vi "Anritsu VNA Set IFBW.vi"(6 "Channel":i8=1 min=1 step=1, 7 "Anritsu VNA":T1, 8 "error in (no error)":errorcluster, 10 "IFBW, Hz (3000)":dbl=3000.0, 11 "VISA Resource Name":refnum<visa-resource-name>) -> (0 "error out":errorcluster, 3 "dup VISA Resource Name":refnum<visa-resource-name>)   [LabVIEW 2011]
doc: "This Vi for the HP8753B Network Analyzer is used to set averaging, smoothing, and the IF bandwidth."
uses:
  TypeDefs/Anritsu VNA Instrument Info.ctl
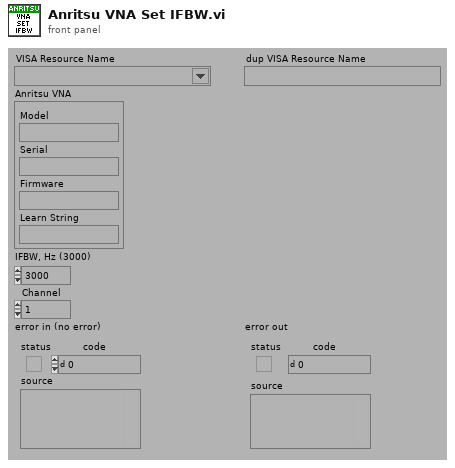
[diagram p1: front panel]
types:
  T1 = typedef "Anritsu VNA Instrument Info.ctl" = cluster{"Model":string, "Serial":string, "Firmware":string, "Learn String":string}
  T2 = typedef "Anritsu VNA Model.ctl" = enum16{"Not Supported", "37XXXX", "MS20XXX", "MS462XX", "MS464XX"}
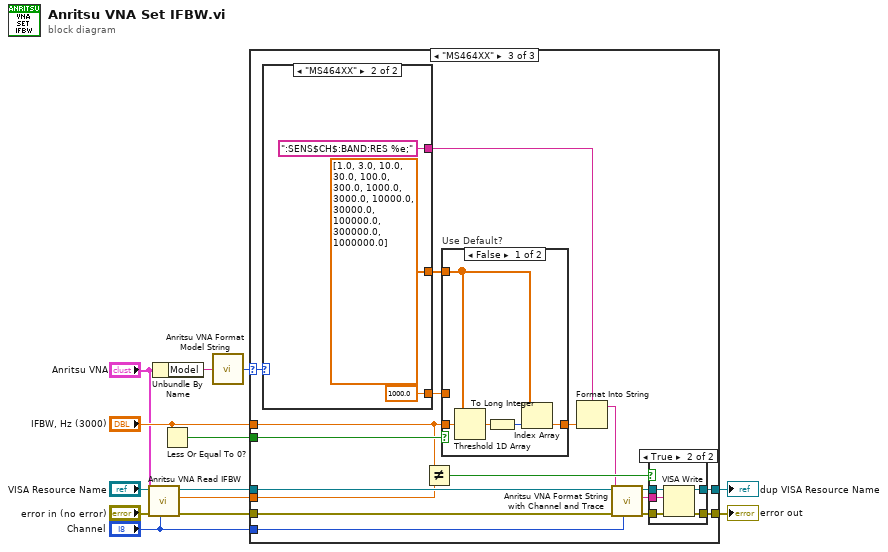
[diagram p0: block diagram]
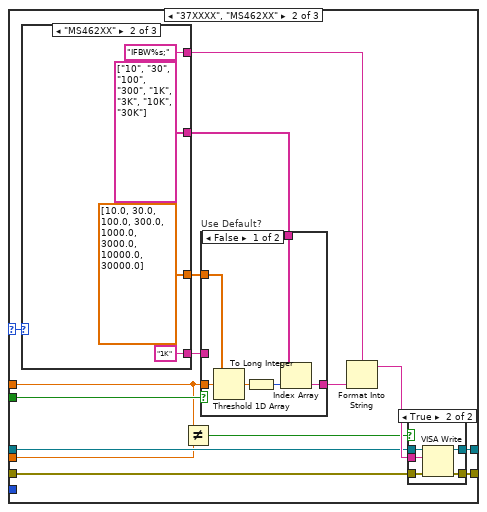
[diagram p3: hidden frame]
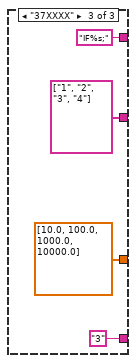
[diagram p6: hidden frame]
diagram:
  n1 = call "Anritsu VNA Read IFBW.vi"("Channel"="Channel", "Anritsu VNA"="Anritsu VNA", "error in (no error)"="error in (no error)", "VISA Resource Name"="VISA Resource Name") -> ("error out"=w8:errorcluster, "IFBW, Hz"=w7:dbl, "dup VISA Resource Name"=w9:refnum<visa-resource-name>)  [unwired: 5 out]
  n2 = Unbundle By Name("Anritsu VNA") -> ("Model"=w3:string)
  n3 = Less Or Equal To 0?(x="IFBW, Hz (3000)") -> (x <= 0?=w5:bool)
  n4 = call "Anritsu VNA Format Model String.vi"("Model"=w3) -> ("Model"=w2:T2)
  n5 = case shown="\"MS464XX\"" w2 {
    selector: w2 -> [_ w21 w60]
    tunnel: [w15 w30 w68] -> w13
    tunnel: [w14 w29 w67] -> w12
    tunnel: w9 -> [w14 w27 w66]
    tunnel: w8 -> [w15 w26 w65]
    tunnel: w7 -> [_ w24 w63]
    tunnel: "IFBW, Hz (3000)" -> [_ w17 w57]
    tunnel: w5 -> [_ w22 w61]
    tunnel: "Channel" -> [_ _ w53]
    frame "Not Supported", "MS20XXX" {
      # "The MS20XXX do not have the ability to set the IFBW."
    }
    frame "37XXXX", "MS462XX" {
      n6 = case shown="\"MS462XX\"" w21 {
        tunnel: [_ dbl[] [10.0, 30.0, 100.0, 300.0, 1000.0, 3000.0, 10000.0, 30000.0] dbl[] [10.0, 100.0, 1000.0, 10000.0]] -> w20
        tunnel: [_ "1K" "3"] -> w19
        tunnel: [_ string[] ["10", "30", "100", "300", "1K", "3K", "10K", "30K"] string[] ["1", "2", "3", "4"]] -> w18
        tunnel: [_ "IFBW%s;" "IF%s;"] -> w16
        frame "Not Supported", "MS20XXX", "MS464XX" {
        }
        frame "MS462XX" {
        }
        frame "37XXXX" {
        }
      }
      n7 = Not Equal?(x=w17, y=w24) -> (x != y?=w25:bool)
      n8 = case "Use Default?" shown="False" w22 {
        tunnel: w20 -> [w35 _]
        tunnel: w17 -> [w33 _]
        tunnel: [w32 w37] -> w23
        tunnel: w19 -> [_ w37]
        tunnel: w18 -> [w31 _]
        frame False {
          n9 = Threshold 1D Array(2:w33, 3:w35) -> (0:w36:dbl)  [unwired: 1 out]
          n10 = To Long Integer(number=w36) -> (32bit integer=w34:i32)
          n11 = Index Array(array=w31, index=w34) -> (element=w32:string)
        }
        frame True {
        }
      }
      n12 = Format Into String(format string=w16, w23) -> (resulting string=w28:string)  [unwired: 2 in, 1 out]
      n13 = case shown="True" w25 {
        tunnel: [w46 w52] -> w30
        tunnel: [w47 w51] -> w29
        tunnel: w28 -> [_ w50]
        tunnel: w27 -> [w47 w49]
        tunnel: w26 -> [w46 w48]
        frame False {
        }
        frame True {
          n14 = VISA Write(VISA resource name=w49, write buffer=w50, error in (no error)=w48) -> (VISA resource name out=w51:refnum<visa-resource-name>, error out=w52:errorcluster)  [unwired: 1 out]
        }
      }
    }
    frame "MS464XX" {
      n15 = case shown="\"MS464XX\"" w60 {
        tunnel: [_ dbl[] [1.0, 3.0, 10.0, 30.0, 100.0, 300.0, 1000.0, 3000.0, 10000.0, 30000.0, 100000.0, 300000.0, 1000000.0]] -> w59
        tunnel: [_ 1000.0] -> w58
        tunnel: [_ ":SENS$CH$:BAND:RES %e;"] -> w56
        frame "Not Supported".."MS462XX" {
        }
        frame "MS464XX" {
        }
      }
      n16 = Not Equal?(x=w57, y=w63) -> (x != y?=w64:bool)
      n17 = case "Use Default?" shown="False" w61 {
        tunnel: w59 -> [w69 _]
        tunnel: w57 -> [w71 _]
        tunnel: [w70 w74] -> w62
        tunnel: w58 -> [_ w74]
        frame False {
          n18 = Threshold 1D Array(2:w71, 3:w69) -> (0:w73:dbl)  [unwired: 1 out]
          n19 = To Long Integer(number=w73) -> (32bit integer=w72:i32)
          n20 = Index Array(array=w69, index=w72) -> (element=w70:dbl)
        }
        frame True {
        }
      }
      n21 = Format Into String(format string=w56, w62) -> (resulting string=w54:string)  [unwired: 2 in, 1 out]
      n22 = call "Anritsu VNA Format String with Channel and Trace.vi"("Channel"=w53, "String"=w54) -> ("String Out"=w55:string)  [unwired: 1 in, 6 out]
      n23 = case shown="True" w64 {
        tunnel: [w78 w84] -> w68
        tunnel: [w79 w83] -> w67
        tunnel: w55 -> [_ w82]
        tunnel: w66 -> [w79 w81]
        tunnel: w65 -> [w78 w80]
        frame False {
        }
        frame True {
          n24 = VISA Write(VISA resource name=w81, write buffer=w82, error in (no error)=w80) -> (VISA resource name out=w83:refnum<visa-resource-name>, error out=w84:errorcluster)  [unwired: 1 out]
        }
      }
    }
  }
  "error out" <- w13
  "dup VISA Resource Name" <- w12
